vi "DWDT_Boolean_Array_to_Digital.vi"(5 "compress data (T)":bool, 8 "error in (no error)":errorcluster, 9 "mode":enum16{"LSB First", "MSB First"}(ring), 10 "delta t":dbl=1000.0 format="%#_6p", 11 "boolean array":bool[][](array[boolean])) -> (0 "error out":errorcluster, 3 "digital waveform":digitalwaveform(waveform)={"t0"=timestamp(0 s since 1904-01-01), "dt"=0.0, "Y"={"transitions"=[], "data"=[]}, "error"={"status"=FALSE, "code"=37421928, "source"=""}})   [LabVIEW 2011]
doc: "Converts a 2D Boolean array to a digital waveform or digital data. You must manually select the polymorphic instance you want to use."
panel:
  in  "Empty Digital WDT":digitalwaveform(waveform)={"t0"=timestamp(0 s since 1904-01-01), "dt"=0.0, "Y"={"transitions"=[], "data"=[]}, "error"={"status"=FALSE, "code"=37421928, "source"=""}}
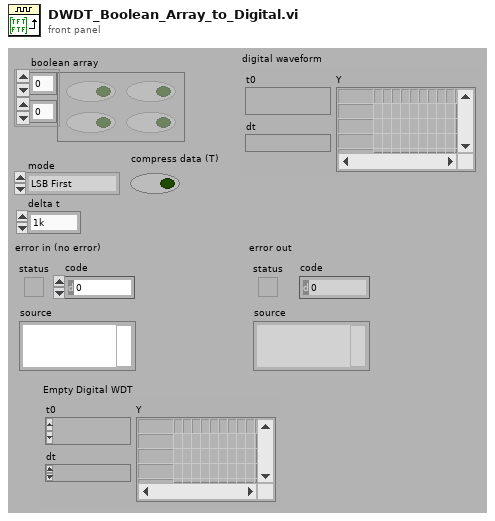
[diagram p1: front panel]
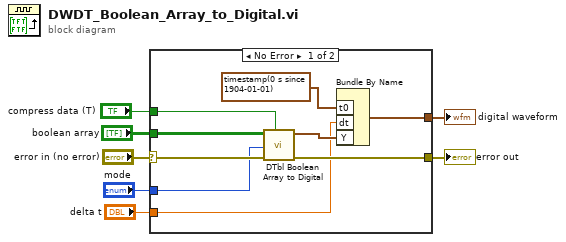
[diagram p0: block diagram]
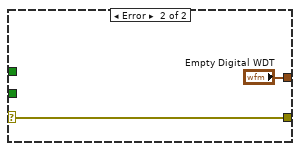
[diagram p2: hidden frame]
diagram:
  n1 = case shown="No Error" "error in (no error)" {
    selector: "error in (no error)" -> [w16 w18]
    tunnel: [w15 w18] -> w7
    tunnel: "boolean array" -> [w14 _]
    tunnel: [w12 "Empty Digital WDT"] -> w4
    tunnel: "mode" -> [w10 _]
    tunnel: "compress data (T)" -> [w9 _]
    tunnel: "delta t" -> [w8 _]
    frame No Error {
      n2 = call <vilib>:"DTbl Boolean Array to Digital.vi"("compress data (T)"=w9, "error in (no error)"=w16, "mode"=w10, "boolean array"=w14) -> ("error out"=w15:errorcluster, "digital data"=w13:digitaldata)  [unwired: 6 in]
      n3 = Bundle By Name("t0"=timestamp(0 s since 1904-01-01), "dt"=w8, "Y"=w13) -> (w12:digitalwaveform)  [unwired: 1 in]
    }
    frame Error {
      # "Incoming Error"
    }
  }
  "digital waveform" <- w4
  "error out" <- w7
